vi "Example Call.vi"() -> ()   [LabVIEW 2015]
uses:
  Input/Input.lvclass
panel:
  out "Error Out":errorcluster
  out "Answer":string
  in  "Greeting":string="Greetings from LabView"
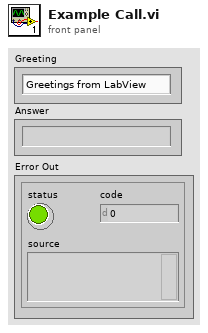
[diagram p1: front panel]
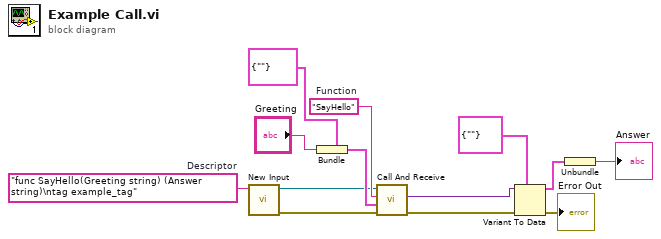
[diagram p0: block diagram]
diagram:
  w6 = "func SayHello(Greeting string) (Answer string)\ntag example_tag"  # Descriptor
  w10 = "SayHello"  # Function
  n1 = call "New Input.vi"("Descriptor"=w6) -> ("error out"=w4:errorcluster, "input out"=w5:refnum<class "Input.lvclass">)  [unwired: 9 in]
  n2 = Bundle(cluster=cluster{"Greeting":string} {"Greeting"=""}, "Greeting"="Greeting") -> (w9:cluster{"Greeting":string})
  n3 = call "Call And Receive.vi"("error in (no error)"=w4, "Parameter"=w9, "Function"=w10, "input in"=w5) -> ("error out"=w7:errorcluster, "Data"=w8:variant)  [unwired: 4 in, 2 out]
  n4 = Variant To Data(error in=w7, type=cluster{"Answer":string} {"Answer"=""}, Variant=w8) -> (data=w11:cluster{"Answer":string}, error out=→"Error Out":errorcluster)
  n5 = Unbundle(w11) -> ("Answer"=→"Answer":string)
